vi "1C.1 Camera - UTMToPixel.vi"(9 "Resolution of camera in pixels":dbl=1384.0, 10 "Width of camera view in meters":dbl=4.648, 11 "Robot UTM Location in":T1) -> (3 "output cluster":cluster{"X":i32, "Y":i32})   [LabVIEW 2011]
uses:
  2-RIO/2 Typedefs/UTM Location.ctl
panel:
  # "Convert UTM to Pixel for 1C camera. \n\nTODO: test edge cases"
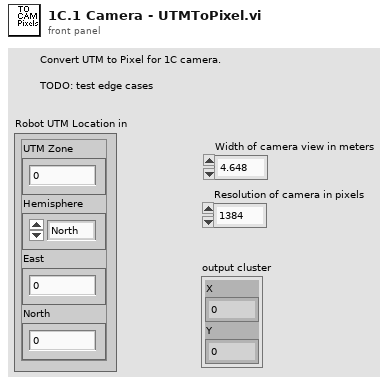
[diagram p1: front panel]
types:
  T1 = typedef "UTM Location.ctl" = cluster{"UTM Zone":dbl, "Hemisphere":enum16{"North", "South"}, "East":dbl, "North":dbl}
  T2 = cluster{"UTM Zone":dbl, "Hemisphere":dbl, "East":dbl, "North":dbl}
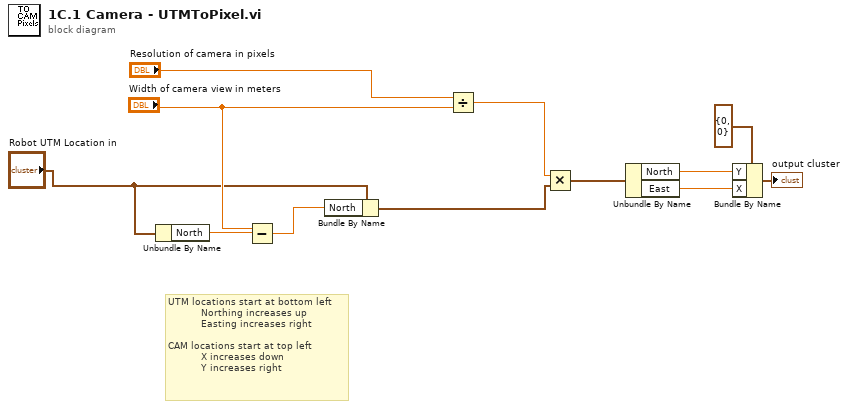
[diagram p0: block diagram]
diagram:
  # "UTM locations start at bottom left\n           Northing increases up\n           Easting increases right\n\nCAM locations start at top left\n           X increases down\n           Y increases right"
  n1 = Unbundle By Name("Robot UTM Location in") -> ("North"=w7:dbl)
  n2 = Subtract(x="Width of camera view in meters", y=w7) -> (x-y=w5:dbl)
  n3 = Bundle By Name(cluster="Robot UTM Location in", "North"=w5) -> (w4:T1)
  n4 = Divide(x="Resolution of camera in pixels", y="Width of camera view in meters") -> (x/y=w11:dbl)
  n5 = Multiply(x=w11, y=w4) -> (x*y=w10:T2)
  n6 = Unbundle By Name(w10) -> ("North"=w9:dbl, "East"=w8:dbl)
  n7 = Bundle By Name(cluster=cluster{"X":i32, "Y":i32} {"X"=0, "Y"=0} ("Point"), "Y"=w9, "X"=w8) -> (→"output cluster":cluster{"X":i32, "Y":i32})
